vi "Write Wärmepumpe.Zustandsgrössen.vi"(8 "error in (no error)":errorcluster, 10 "Wärmepumpe.Zustandsgrössen":T1, 11 "Wärmepumpe in":refnum<class "Wärmepumpe.lvclass">) -> (0 "error out":errorcluster, 3 "Wärmepumpe out":refnum<class "Wärmepumpe.lvclass">)   [LabVIEW 2016, in "Wärmepumpe.lvclass"]
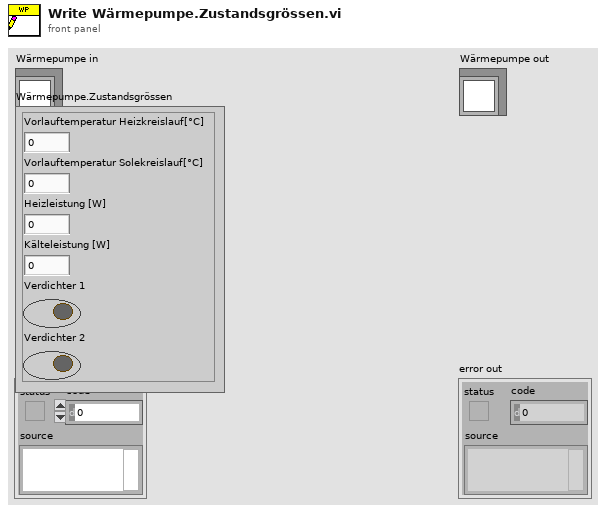
[diagram p1: front panel]
types:
  T1 = typedef "Wärmepumpe.lvclass/Wärmepumpe.Zustandsgrössen.ctl" = cluster{"Vorlauftemperatur Heizkreislauf[°C]":dbl, "Vorlauftemperatur Solekreislauf[°C]":dbl, "Heizleistung [W]":dbl, "Kälteleistung [W]":dbl, "Verdichter 1":bool, "Verdichter 2":bool}
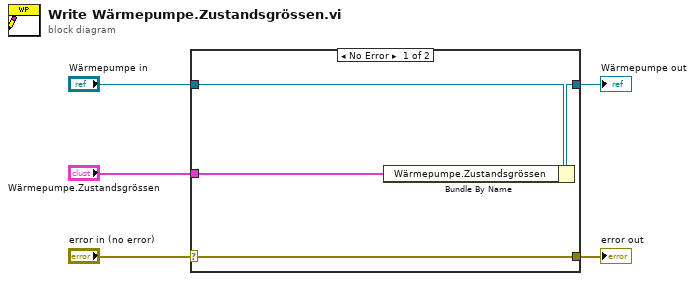
[diagram p0: block diagram]
diagram:
  n1 = case shown="No Error" "error in (no error)" {
    selector: "error in (no error)" -> [w9 w10]
    tunnel: [w9 w10] -> w4
    tunnel: [w7 w11] -> w2
    tunnel: "Wärmepumpe in" -> [w8 w11]
    tunnel: "Wärmepumpe.Zustandsgrössen" -> [w6 _]
    frame No Error {
      n2 = Bundle By Name(cluster=w8, "Wärmepumpe.Zustandsgrössen"=w6) -> (w7:refnum<class "Wärmepumpe.lvclass">)
    }
    frame Error {
    }
  }
  "error out" <- w4
  "Wärmepumpe out" <- w2
